vi "Simplex-AO.vi"(3 "Initial Simplex Guess":path=path "C:/Users/Mlodzianoski/Desktop/Microscope 2 Labview Programs/VIs/DM/Mike/FitVal_ZMode_Depth_Corr_April5-2017_Temp.txt", 5 "Current Z":dbl=0.096933, 6 "DM Function":T1=enum."Simplex Correction", 8 "Cycle #":u16, 9 "Step #":u16, 13 "Initial Z":dbl=0.104477, 14 "Use Coverslip Postion":bool=TRUE, 15 "Coverslip Position":dbl=0.103603) -> (19 "Xmin_final":dbl[](array[numeric]))   [LabVIEW 2015]
uses:
  subvis/DM Function_v2.ctl
panel:
  in  "Vertical Coma":bool
  in  "Horizontal Coma":bool
  in  "Vertical Astigmatism":bool
  in  "Oblique Astigmatism":bool
  in  "2nd Spherical Aberration":bool
  in  "1st  Spherical Aberration":bool
  in  "a":dbl=-5e-05 format="%#_13g"
  in  "b":dbl=0.0253 format="%#_13g"
  in  "c":dbl=1.5 format="%#_13g"
  in  "Use Adaptive Astigmatism":bool
  in  "Zernike Modes 3":i32[](array[numeric])
  out "camera sub-readout":u16[][](graph)
  out "current n":i32
  in  "Use Cursor":bool
  in  "boxsize":i32=200
  in  "Use Simplex Results":bool
  in  "Zernike Modes 1":i32[](array[numeric])=[11, 22]
  in  "Zernike Modes 2":i32[](array[numeric])=[5, 6, 7, 8]
  out "Original Simplex Input":dbl[](array[numeric])
  out "Imaging Astigmatism Values":string[](array[string])
  in  "N":i32=40
  out "Tolerance Met":bool
  in  "parray Tolerance\nThreshold":dbl=0.0005
  in  "x input Tolerance\nThreshold":dbl=0.03
  out "xr":dbl[](array[numeric])
  out "parray":dbl[](array[numeric])
  out "Simplex Amplitude":dbl[][](array[numeric])
  in  "indM":i32
  in  "pin":dbl format="%#_13g"
  out "xin":dbl[](array[numeric])
  out "xmax":dbl[](array[numeric])
  out "centroid":dbl[](array[numeric])
  out "xmin":dbl[](array[numeric])
  out "pmax_ind":i32
  out "pmin_ind":i32
  out "psmax":dbl
  out "pmax":dbl
  out "pmin":dbl
  out "pvalr":dbl
  out "camera readout":u16[][](graph)
  # "Adaptive  Astigmatism"
  # "Inputs from \nImaging Program"
  # "Depth Settings"
  # "2nd order polynomial  values from curve fit to data in S. Fig 13"
  # "Aberration Selector"
  # "Column number corresponds to Zernike Mode, value is magnitude of DM."
  # "Current Vertices"
  # "Simplex vertices (updated to show best values)"
  # "Metric pval\ncorresponding \ncurrent set  of \nvertices in \nSimplex \nAmplitude."
  # "Current optimal simplex value"
  # "Final (optimized) simplex values."
  # "Original Simplex Inputs"
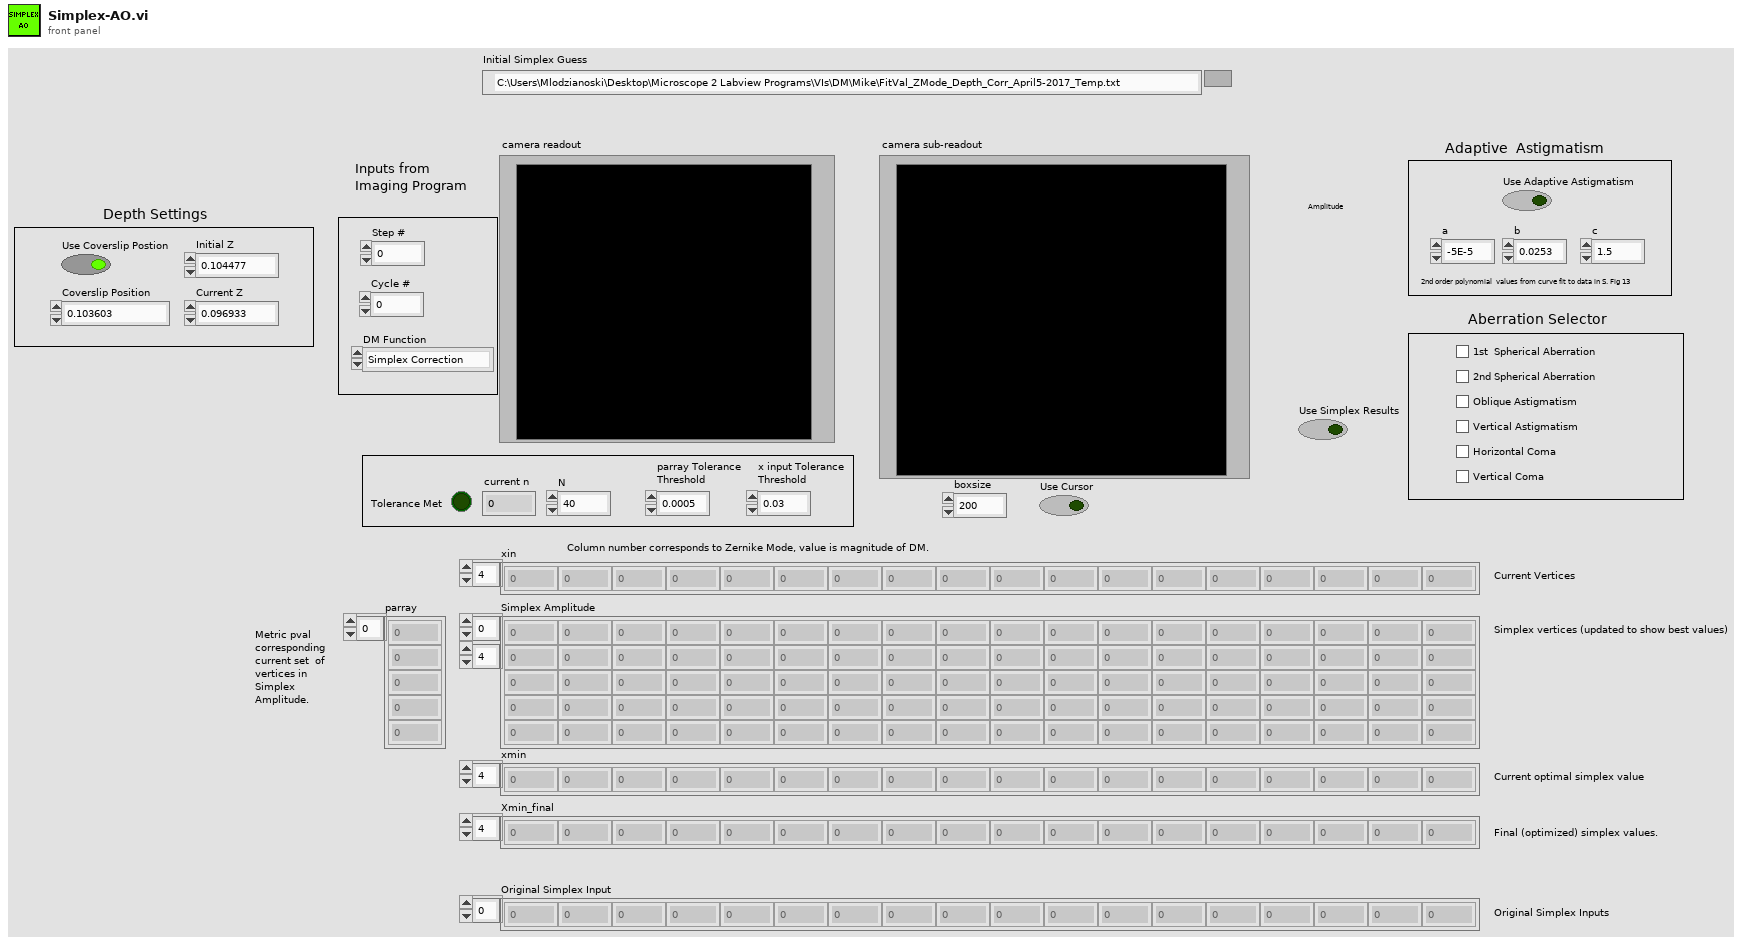
[diagram p1: front panel]
types:
  T1 = typedef "DM Function_v2.ctl" = enum16{"Find Mirror Modes", "Aberration Scan", "Live Aberration Correction", "Idle", "Simplex Correction"}
  T2 = typedef "AbberationControl.ctl" = cluster{"Abberations":dbl[][], "Modes":i32[], "Flat":dbl[], "Abberations ID":string[][]}
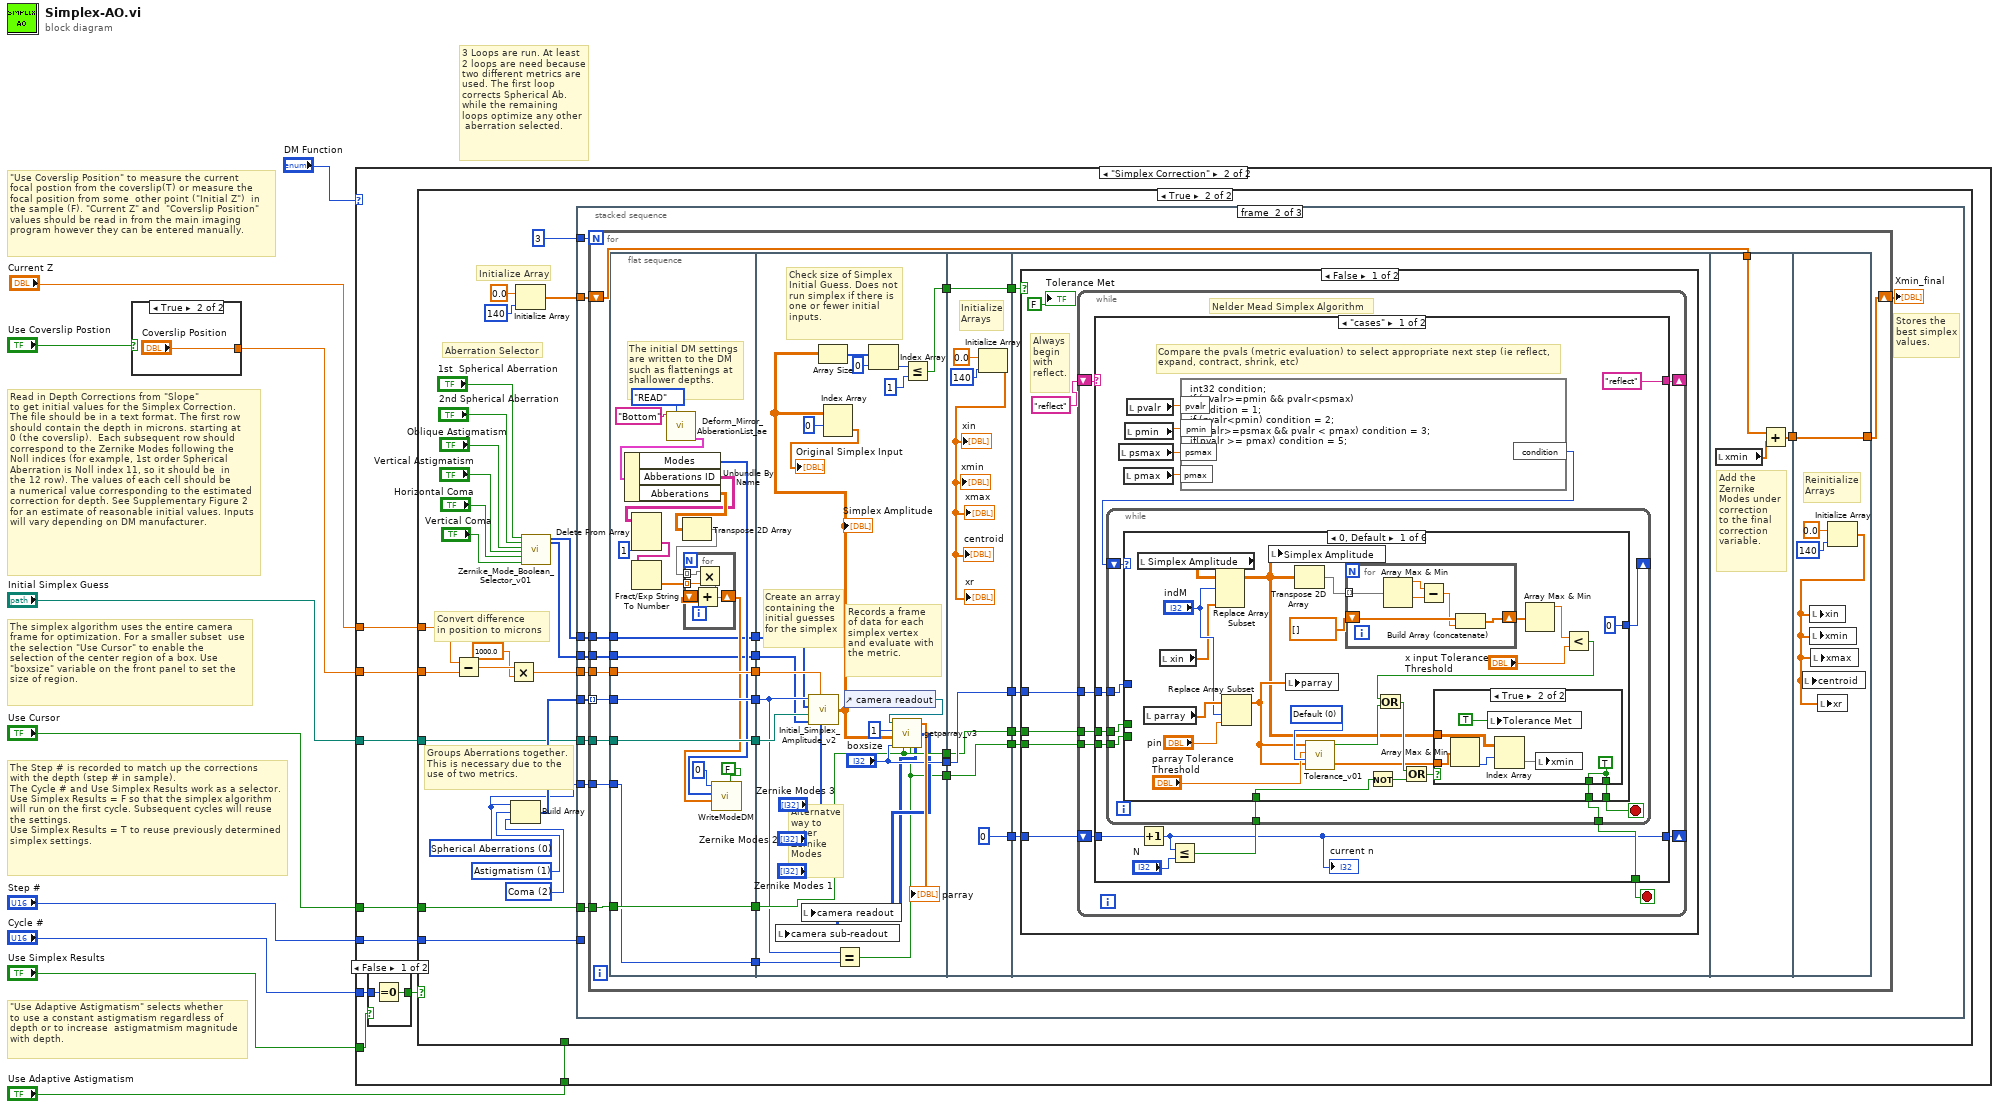
[diagram p0: block diagram]
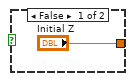
[diagram p2: hidden frame]
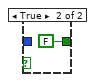
[diagram p4: hidden frame]
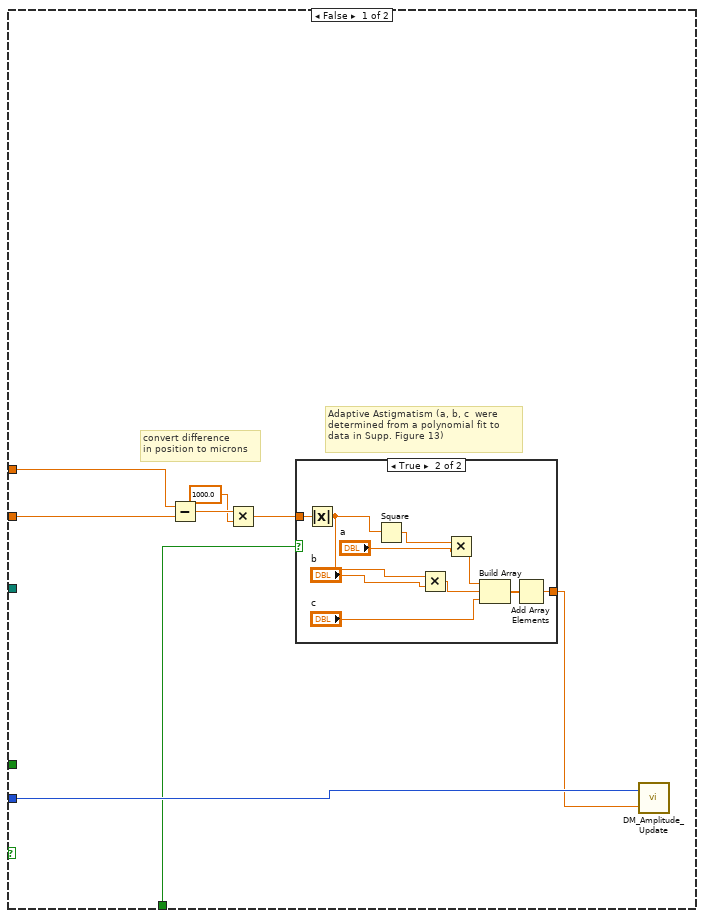
[diagram p5: hidden frame]
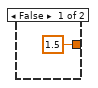
[diagram p6: hidden frame]
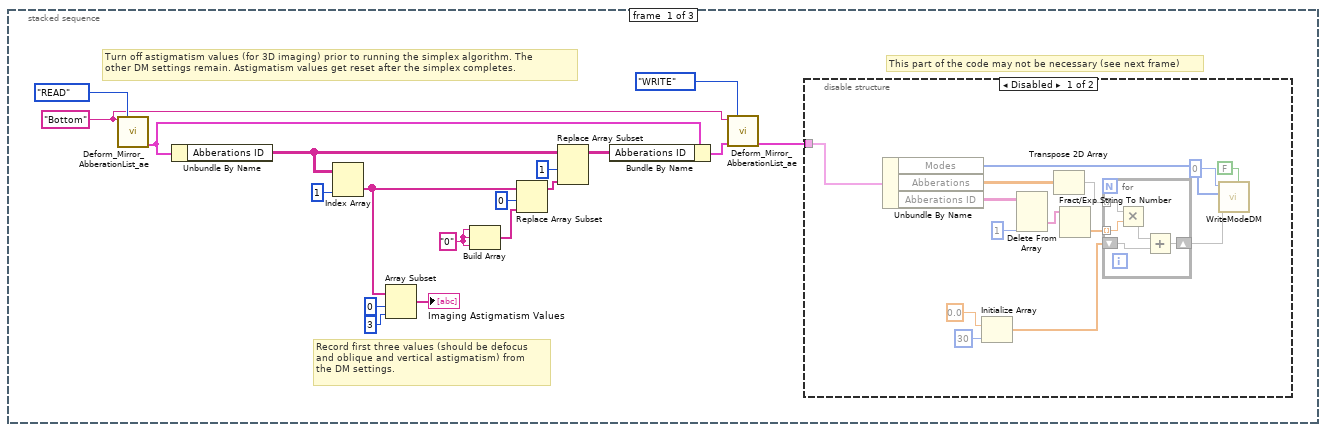
[diagram p7: hidden frame]
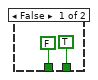
[diagram p9: hidden frame]
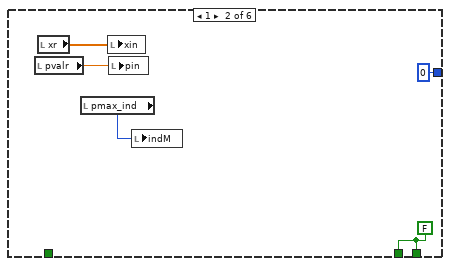
[diagram p10: hidden frame]
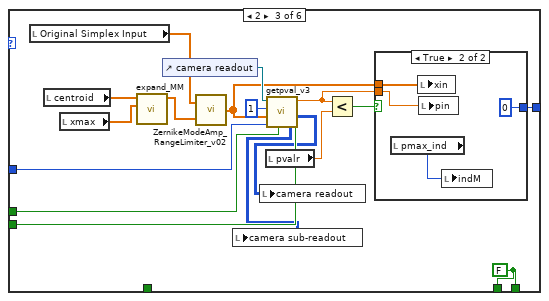
[diagram p11: hidden frame]
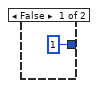
[diagram p12: hidden frame]
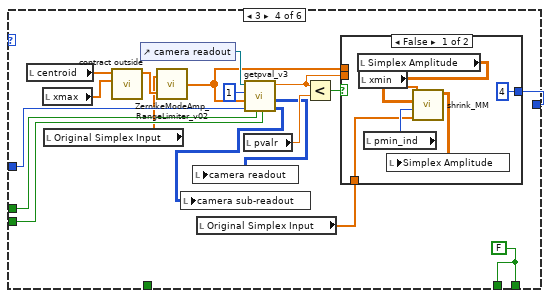
[diagram p13: hidden frame]
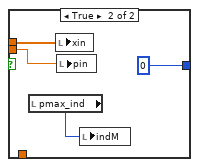
[diagram p14: hidden frame]
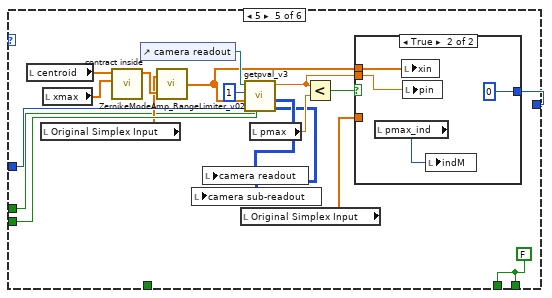
[diagram p15: hidden frame]
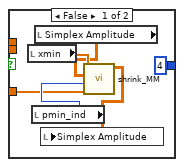
[diagram p16: hidden frame]
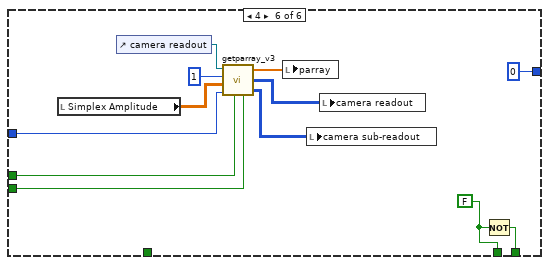
[diagram p17: hidden frame]
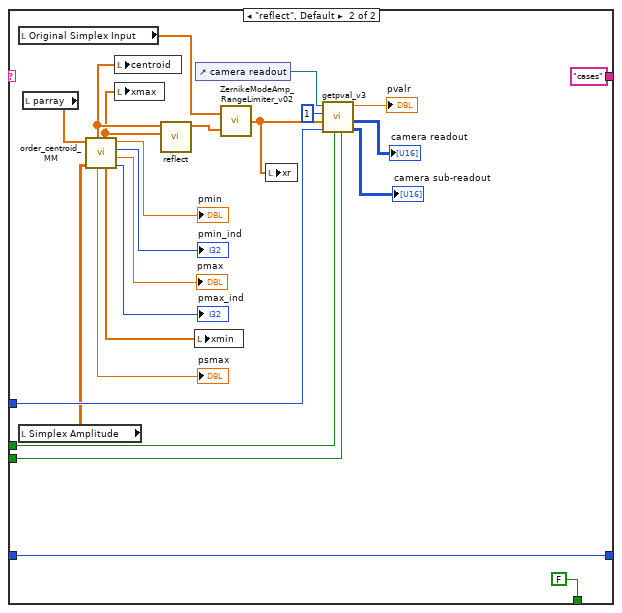
[diagram p18: hidden frame]
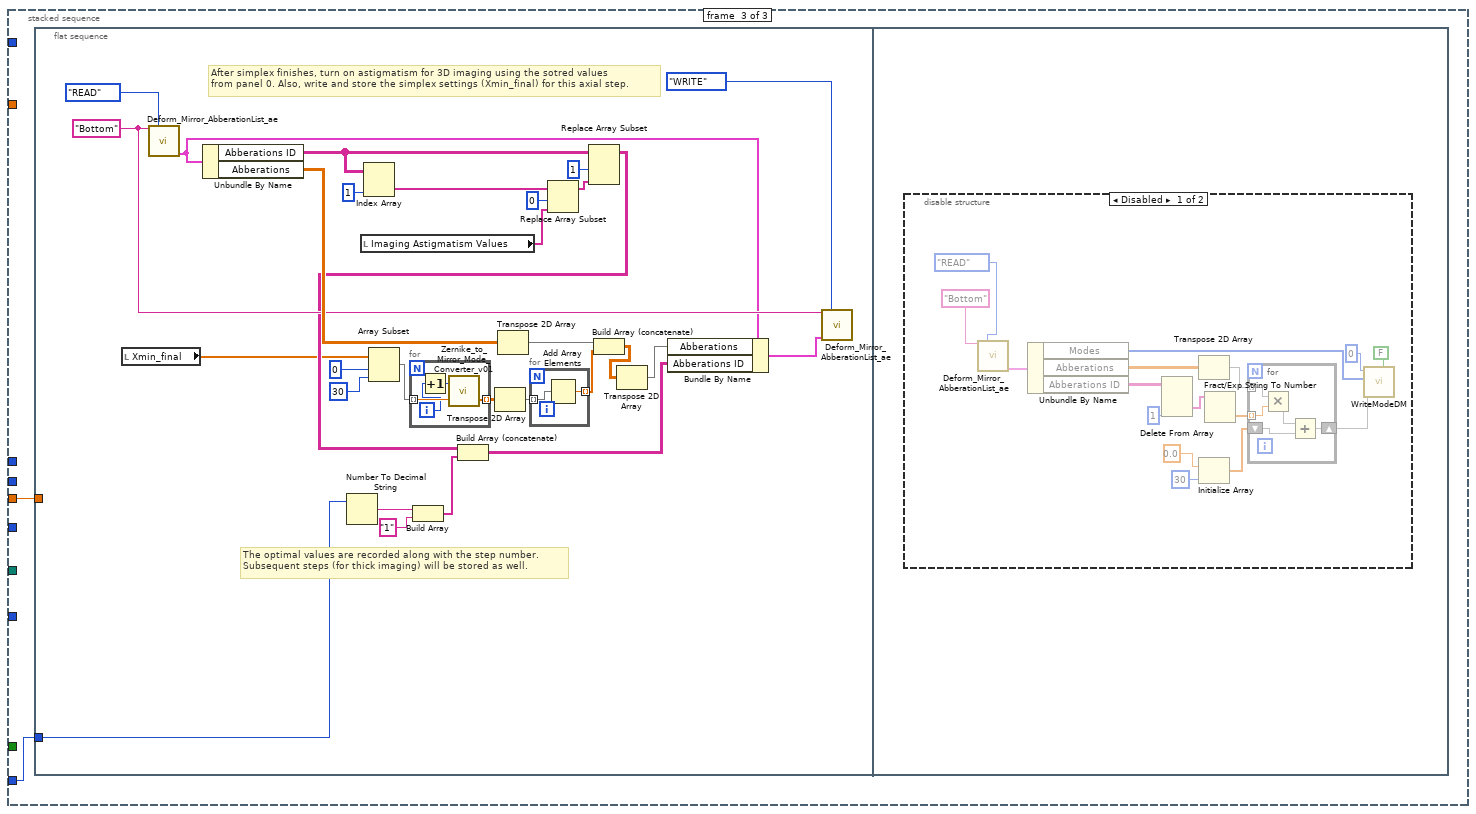
[diagram p20: hidden frame]
diagram:
  # "3 Loops are run. At least\n2 loops are need because\ntwo different metrics are\nused. The first loop \ncorrects Spherical Ab. \nwhile the remaining \nloops optimize any other\n aberration selected."
  # "\"Use Adaptive Astigmatism\" selects whether\nto use a constant astigmatism regardless of \ndepth or to increase  astigmatmism magnitude\nwith depth."
  # "The Step # is recorded to match up the corrections\nwith the depth (step # in sample).\nThe Cycle # and Use Simplex Results work as a selector.\nUse Simplex Results = F so that the simplex algorithm\nwill run on the first cycle. Subsequent cycles will reuse \nthe settings. \nUse Simplex Results = T to reuse previously determined\nsimplex settings."
  # "The simplex algorithm uses the entire camera\nframe for optimization. For a smaller subset  use\nthe selection \"Use Cursor\" to enable the\nselection of the center region of a box. Use\n\"boxsize\" variable on the front panel to set the \nsize of region."
  # "\"Use Coverslip Position\" to measure the current \nfocal postion from the coverslip(T) or measure the\nfocal position from some  other point (\"Initial Z\")  in \nthe sample (F). \"Current Z\" and  \"Coverslip Position\" \nvalues should be read in from the main imaging \nprogram however they can be entered manually."
  # "Read in Depth Corrections from \"Slope\"\nto get initial values for the Simplex Correction.\nThe file should be in a text format. The first row\nshould contain the depth in microns. starting at \n0 (the coverslip).  Each subsequent row should \ncorrespond to the Zernike Modes following the \nNoll indices (for example, 1st order Spherical\nAberration is Noll index 11, so it should be  in \nthe 12 row). The values of each cell should be \na numerical value corresponding to the estimated\ncorrection for depth. See Supplementary Figure 2\nfor an estimate of reasonable initial values. Inputs\nwill vary depending on DM manufacturer."
  n1 = case shown="True" "Use Coverslip Postion" {
    tunnel: ["Initial Z" "Coverslip Position"] -> w10
    frame False {
    }
    frame True {
    }
  }
  n2 = case shown="\"Simplex Correction\"" "DM Function" {
    tunnel: "Current Z" -> [_ w21]
    tunnel: w10 -> [_ w20]
    tunnel: "Initial Simplex Guess" -> [_ w19]
    tunnel: "Step #" -> [_ w18]
    tunnel: "Cycle #" -> [_ w17]
    tunnel: "Use Simplex Results" -> [_ w14]
    tunnel: "Use Cursor" -> [_ w15]
    tunnel: "Use Adaptive Astigmatism" -> [_ w13]
    frame "Idle", Default {
    }
    frame "Simplex Correction" {
      n3 = case shown="False" w14 {
        tunnel: w17 -> [w23 _]
        tunnel: [w22 FALSE] -> w16
        frame False {
          n4 = Equal To 0?(x=w23) -> (x = 0?=w22:bool)
        }
        frame True {
        }
      }
      n5 = case shown="True" w16 {
        tunnel: w21 -> [w28 w65]
        tunnel: w20 -> [w27 w64]
        tunnel: w19 -> [_ w45]
        tunnel: w18 -> [w32 w57]
        tunnel: w15 -> [_ w56]
        tunnel: w13 -> [w26 _]
        frame False {
          # "Adaptive Astigmatism (a, b, c  were\ndetermined from a polynomial fit to \ndata in Supp. Figure 13)"
          # "convert difference \nin position to microns"
          n6 = Subtract(x=w28, y=w27) -> (x-y=w30:dbl)
          n7 = Multiply(x=w30, y=1000.0) -> (x*y=w31:dbl)
          n8 = case shown="True" w26 {
            tunnel: w31 -> [_ w43]
            tunnel: [1.5 ("y") w38] -> w25
            frame False {
            }
            frame True {
              n9 = Absolute Value(x=w43) -> (abs(x)=w41:dbl)
              n10 = Square(x=w41) -> (x^2=w42:dbl)
              n11 = Multiply(x=w41, y="b") -> (x*y=w37:dbl)
              n12 = Multiply(x=w42, y="a") -> (x*y=w40:dbl)
              n13 = Build Array(w40, w37, "c") -> (w39:dbl[])
              n14 = Add Array Elements(numeric array=w39) -> (sum=w38:dbl)
            }
          }
          n15 = call "DM_Amplitude_Update.vi"("Adaptive Astigmatism Value"=w25, "Step #"=w32) -> ()  [unwired: 1 in]
        }
        frame True {
          w54 = u16 2 items=["Spherical Aberrations", "Astigmatism", "Coma"] ("Aberration Correction Choice")
          w55 = u16 1 items=["Spherical Aberrations", "Astigmatism", "Coma"] ("Aberration Correction Choice")
          w44 = u16 0 items=["Spherical Aberrations", "Astigmatism", "Coma"] ("Aberration Correction Choice")
          # "Groups Aberrations together.\nThis is necessary due to the \nuse of two metrics."
          # "Aberration Selector"
          # "Initialize Array"
          # "Convert difference \nin position to microns"
          n16 = Subtract(x=w65, y=w64) -> (x-y=w67:dbl)
          n17 = Multiply(x=w67, y=1000.0) -> (x*y=w63:dbl)
          n18 = Build Array(w44, w55, w54) -> (w61:u16[])
          n19 = Initialize Array(0.0 ("element"), 140 ("dimension size")) -> (w58:dbl[])
          n20 = call "Zernike_Mode_Boolean_Selector_v01.vi"("1st  Spherical Aberration"="1st  Spherical Aberration", "2nd Spherical Aberration"="2nd Spherical Aberration", "Oblique Astigmatism"="Oblique Astigmatism", "Vertical Astigmatism"="Vertical Astigmatism", "Horizontal Coma"="Horizontal Coma", "Vertical Coma"="Vertical Coma") -> ("ZM 1"=w47:i32[], "ZM 2"=w46:i32[])  [unwired: 12 in]
          n21 = stacked-sequence {
            tunnel: w63 -> [_ w114 w401]
            tunnel: w45 -> [_ w113 _]
            tunnel: 3 -> [_ w112 _]
            tunnel: w58 -> [_ w109 _]
            tunnel: w61 -> [_ w111 _]
            tunnel: w57 -> [_ _ w402]
            tunnel: w56 -> [_ w108 _]
            tunnel: w44 -> [_ w107 _]
            tunnel: w47 -> [_ w106 _]
            tunnel: w46 -> [_ w105 _]
            frame #0 {
              w71 = "0"
              w84 = "Bottom" ("Mirror ID")
              # "This part of the code may not be necessary (see next frame)"
              # "Turn off astigmatism values (for 3D imaging) prior to running the simplex algorithm. The \nother DM settings remain. Astigmatism values get reset after the simplex completes."
              # "Record first three values (should be defocus \nand oblique and vertical astigmatism) from \nthe DM settings."
              n22 = call "Deform_Mirror_AbberationList_ae.vi"("Mirror ID"=w84, "Enum"=enum16{"WRITE", "READ"}."READ") -> ("Abberation Cluster Out"=w81:T2)  [unwired: 12 in, 1 out]
              n23 = Unbundle By Name(w81) -> ("Abberations ID"=w75:string[][])
              n24 = Index Array(array=w75, index (col)=1 ("disabled index (col)")) -> (element=w76:string[])  [unwired: 1 in]
              n25 = Array Subset(array=w76, index=0, length=3) -> (→"Imaging Astigmatism Values":string[])
              n26 = Build Array(w71, w71, w71) -> (w70:string[])
              n27 = Replace Array Subset(array=w76, new element=w70, index=0 ("index (row)")) -> (w74:string[])
              n28 = Replace Array Subset(array=w75, new element=w74, index (col)=1 ("disabled index (col)")) -> (w72:string[][])  [unwired: 1 in]
              n29 = Bundle By Name(cluster=w81, "Abberations ID"=w72) -> (w82:T2)
              n30 = call "Deform_Mirror_AbberationList_ae.vi"("Mirror ID"=w84, "Enum"=enum16{"WRITE", "READ"}."WRITE", "Abberation Cluster In"=w82) -> ("Abberation Cluster Out"=w68:T2)  [unwired: 11 in, 1 out]
              n31 = disable-structure shown="Disabled" {
                disable-tunnel: w68 -> [w89 _]
                frame Disabled {
                  n32 = Unbundle By Name(w89) -> ("Modes"=w92:i32[], "Abberations"=w97:dbl[][], "Abberations ID"=w96:string[][])
                  n33 = Initialize Array(0.0 ("element"), 30 ("dimension size")) -> (w86:dbl[])
                  n34 = Delete From Array(array=w96, index (col)=1 ("index")) -> (deleted portion=w94:string[])  [unwired: 2 in, 1 out]
                  n35 = Transpose 2D Array(2D array=w97) -> (transposed array=w98:dbl[][])
                  n36 = Fract/Exp String To Number(string=w94) -> (number=w99:dbl[])  [unwired: 3 in, 1 out]
                  n37 = for {
                    shift-right: [w100] -> w93
                    shift-left: w86 -> [w102]
                    tunnel: w98 -> [w104] mode=indexing
                    tunnel: w99 -> [w103] mode=indexing
                    n38 = Multiply(x=w104, y=w103) -> (x*y=w101:dbl[])
                    n39 = Add(x=w101, y=w102) -> (x+y=w100:dbl[])
                  }
                  n40 = call "WriteModeDM.vi"("ClearV"=FALSE, "Amplitudes"=w93, "Modes"=w92, "Device"=0) -> ()  [unwired: 7 in, 1 out]
                }
                frame Enabled {
                }
              }
            }
            frame #1 {
              # "Stores the\nbest simplex\nvalues."
              n41 = for {
                N: w112 -> [_]
                tunnel: w114 -> [w140]
                tunnel: w113 -> [w139]
                tunnel: w111 -> [w138] mode=indexing
                shift-right: [w137] -> w110
                shift-left: w109 -> [w131]
                tunnel: w108 -> [w126]
                tunnel: w107 -> [w120]
                tunnel: w106 -> [w117]
                tunnel: w105 -> [w115]
                n42 = flat-sequence {
                  tunnel: w138 -> [w158]
                  tunnel: w139 -> [w159]
                  tunnel: w140 -> [w160]
                  tunnel: [w160] -> w130
                  tunnel: [w159] -> w129
                  tunnel: [w158] -> w128
                  tunnel: [w145] -> w127
                  tunnel: w126 -> [w145]
                  tunnel: [w144] -> w121
                  tunnel: w120 -> [w144]
                  tunnel: [w142] -> w118
                  tunnel: w117 -> [w142]
                  tunnel: [w141] -> w116
                  tunnel: w115 -> [w141]
                  tunnel: [w170] -> w135
                  tunnel: ["boxsize"] -> w133
                  tunnel: w130 -> [w185]
                  tunnel: w129 -> [w184]
                  tunnel: w128 -> [w172]
                  tunnel: w127 -> [w180]
                  tunnel: [w180] -> w124
                  tunnel: [w175] -> w122
                  tunnel: w121 -> [w171]
                  tunnel: w118 -> [w168]
                  tunnel: w116 -> [w167]
                  tunnel: w135 -> [w196]
                  tunnel: [w196] -> w134
                  tunnel: w133 -> [w195]
                  tunnel: [w195] -> w132
                  tunnel: [w191] -> w125
                  tunnel: w124 -> [w191]
                  tunnel: [w190] -> w123
                  tunnel: w122 -> [w190]
                  tunnel: [0] -> w119
                  tunnel: w134 -> [w201]
                  tunnel: w132 -> [w200]
                  tunnel: w125 -> [w199]
                  tunnel: w123 -> [w198]
                  tunnel: w119 -> [w197]
                  tunnel: w131 -> [w394]
                  tunnel: [w395] -> w136
                  tunnel: [w400] -> w137
                  tunnel: w136 -> [w400]
                  frame #0 {
                    # "The initial DM settings\nare written to the DM\nsuch as flattenings at \nshallower depths."
                    n43 = call "Deform_Mirror_AbberationList_ae.vi"("Mirror ID"="Bottom", "Enum"=enum16{"WRITE", "READ"}."READ") -> ("Abberation Cluster Out"=w155:T2)  [unwired: 12 in, 1 out]
                    n44 = Unbundle By Name(w155) -> ("Modes"=w146:i32[], "Abberations ID"=w149:string[][], "Abberations"=w150:dbl[][])
                    n45 = Delete From Array(array=w149, index (col)=1 ("index")) -> (deleted portion=w153:string[])  [unwired: 2 in, 1 out]
                    n46 = Fract/Exp String To Number(string=w153) -> (number=w154:dbl[])  [unwired: 3 in, 1 out]
                    n47 = Transpose 2D Array(2D array=w150) -> (transposed array=w151:dbl[][])
                    n48 = for {
                      shift-right: [w163] -> w147
                      shift-left: _ -> [w165]
                      tunnel: w151 -> [w162] mode=indexing
                      tunnel: w154 -> [w161] mode=indexing
                      n49 = Multiply(x=w162, y=w161) -> (x*y=w164:dbl[])
                      n50 = Add(x=w164, y=w165) -> (x+y=w163:dbl[])
                    }
                    n51 = call "WriteModeDM.vi"("ClearV"=FALSE, "Amplitudes"=w147, "Modes"=w146, "Device"=0) -> ()  [unwired: 7 in, 1 out]
                  }
                  frame #1 {
                    # "Alternatve\nway to \nenter \nZernike\nModes"
                    # "Records a frame\nof data for each \nsimplex vertex \nand evaluate with \nthe metric."
                    # "Check size of Simplex \nInitial Guess. Does not\nrun simplex if there is  \none or fewer initial\ninputs."
                    # "Create an array\ncontaining the \ninitial guesses \nfor the simplex"
                    n52 = call "Initial_Simplex_Amplitude_v2.vi"("Zernike Modes 3"="Zernike Modes 3", "Depth (um)"=w185, "Zernike Modes 2"=w167, "Slope"=w184, "Zernike Modes 1"=w168, "Aberration Correction Choice"=w172) -> ("Initial Simplex Amplitude"=w166:dbl[][])
                    "Simplex Amplitude" <- w166
                    n53 = Array Size(array=w166) -> (size(s)=w179:i32[])
                    n54 = Index Array(array=w166, index (row)=0) -> (element=→"Original Simplex Input":dbl[])  [unwired: 1 in]
                    n55 = Equal?(x=w172, y=w171) -> (x = y?=w170:bool)
                    n56 = control-ref of="camera readout"() -> (w186:refnum<vi>)
                    n57 = Index Array(array=w179, index=0) -> (element=w177:i32)
                    n58 = call "getparray_v3.vi"("IntensityGraph in"=w186, "Metric Choice"=w170, "Frames number"=1, "update M"=w166, "Use Cursor"=w180, "boxsize"="boxsize") -> ("Array"=→"parray":dbl[], "subarray"=w174:u16[][], "sub subarray"=w173:u16[][])
                    n59 = local write "camera sub-readout"(w173) -> ()
                    n60 = local write "camera readout"(w174) -> ()
                    n61 = Less Or Equal?(x=w177, y=1) -> (x <= y?=w175:bool)
                  }
                  frame #2 {
                    # "Initialize\nArrays"
                    n62 = Initialize Array(0.0 ("element"), 140 ("dimension size")) -> (→"centroid" →"xmax" →"xmin" →"xr" →"xin":dbl[])
                  }
                  frame #3 {
                    n63 = case shown="False" w198 {
                      tunnel: w201 -> [w206 _]
                      tunnel: w200 -> [w205 _]
                      tunnel: w199 -> [w204 _]
                      tunnel: w197 -> [w203 _]
                      frame False {
                        # "Always\nbegin \nwith\nreflect."
                        n64 = while {
                          shift-right: [w212] -> _
                          shift-left: "reflect" -> [w215]
                          tunnel: w205 -> [w214]
                          tunnel: w206 -> [w213]
                          tunnel: w204 -> [w210]
                          shift-right: [w208] -> _
                          shift-left: w203 -> [w209]
                          stop <- w211 stop-if-true
                          # "Nelder Mead Simplex Algorithm"
                          n65 = case shown="\"cases\"" w215 {
                            tunnel: w214 -> [w223 w390]
                            tunnel: w213 -> [w222 w389]
                            tunnel: ["reflect" "cases"] -> w212
                            tunnel: [w221 FALSE] -> w211
                            tunnel: w210 -> [w220 w372]
                            tunnel: w209 -> [w217 w370]
                            tunnel: [w216 w370] -> w208
                            frame "cases" {
                              # "Compare the pvals (metric evaluation) to select appropriate next step (ie reflect, \nexpand, contract, shrink, etc)"
                              n66 = local read "psmax"() -> (w227:dbl)
                              n67 = local read "pmax"() -> (w226:dbl)
                              n68 = local read "pmin"() -> (w228:dbl)
                              n69 = local read "pvalr"() -> (w229:dbl)
                              n70 = Increment(x=w217) -> (x+1=w216:i32)
                              "current n" <- w216
                              n71 = Less Or Equal?(x=w216, y="N") -> (x <= y?=w218:bool)
                              n72 = formula code="int32 condition;\nif (pvalr>=pmin && pvalr<psmax)\n condition = 1;\nif (pvalr<pmin) condition = 2;\nif(pvalr>=psmax && pvalr < pmax) condition = 3;\nif(pvalr >= pmax) condition = 5;"("pvalr"=w229, "pmin"=w228, "psmax"=w227, "pmax"=w226) -> ("condition"=w225:i32)
                              n73 = while {
                                tunnel: w223 -> [w236]
                                tunnel: w222 -> [w235]
                                shift-right: [w234] -> _
                                shift-left: w225 -> [w237]
                                tunnel: [w231] -> w221
                                tunnel: w218 -> [w232]
                                tunnel: w220 -> [w230]
                                stop <- w233 stop-if-true
                                n74 = case shown="0, Default" w237 {
                                tunnel: w236 -> [_ _ w294 w313 w341 w368]
                                tunnel: w235 -> [_ _ w291 w312 w340 w366]
                                tunnel: [0 0 w288 w308 w336 0] -> w234
                                tunnel: [w247 w275 w285 w307 w335 w363] -> w233
                                tunnel: w232 -> [w246 _ _ _ _ _]
                                tunnel: [w242 w275 w285 w307 w335 w362] -> w231
                                tunnel: w230 -> [_ _ w281 w303 w331 w360]
                                frame 0, Default {
                                w254 = u16 0 items=["Default", "Five Best p-values"] ("Ring")
                                n75 = local read "Simplex Amplitude"() -> (w240:dbl[][])
                                n76 = local read "parray"() -> (w258:dbl[])
                                n77 = local read "xin"() -> (w238:dbl[])
                                n78 = Replace Array Subset(array=w240, new element=w238, index (row)="indM") -> (w239:dbl[][])  [unwired: 1 in]
                                n79 = Replace Array Subset(array=w258, new element="pin", index="indM") -> (w241:dbl[])
                                n80 = local write "Simplex Amplitude"(w239) -> ()
                                n81 = local write "parray"(w241) -> ()
                                n82 = Transpose 2D Array(2D array=w239) -> (transposed array=w259:dbl[][])
                                n83 = call "Tolerance_v01.vi"("Ring"=w254, "Tolerance Threshold"="parray Tolerance\nThreshold", "parray"=w241) -> ("Boolean"=w249:bool)  [unwired: 8 in]
                                n84 = for {
                                tunnel: w259 -> [w274] mode=indexing
                                shift-right: [w271] -> w251
                                shift-left: dbl[] [] -> [w270]
                                n85 = Array Max & Min(array=w274) -> (max value=w273:dbl, min value=w272:dbl)  [unwired: 2 out]
                                n86 = Subtract(x=w273, y=w272) -> (x-y=w269:dbl)
                                n87 = Build Array (concatenate)(w270, w269) -> (w271:dbl[])
                                }
                                n88 = Not(x=w246) -> (.not. x?=w245:bool)
                                n89 = Array Max & Min(array=w251) -> (max value=w252:dbl)  [unwired: 3 out]
                                n90 = Less?(x=w252, y="x input Tolerance\nThreshold") -> (x < y?=w248:bool)
                                n91 = Or(x=w248, y=w249) -> (x .or. y?=w244:bool)
                                n92 = Or(x=w244, y=w245) -> (x .or. y?=w243:bool)
                                n93 = case shown="True" w243 {
                                tunnel: w241 -> [_ w266]
                                tunnel: w239 -> [_ w265]
                                tunnel: [TRUE w263] -> w247
                                tunnel: [FALSE w263] -> w242
                                frame False {
                                }
                                frame True {
                                w263 = TRUE
                                n94 = Array Max & Min(array=w266) -> (min index (indices)=w267:i32)  [unwired: 3 out]
                                n95 = local write "Tolerance Met"(TRUE) -> ()
                                n96 = Index Array(array=w265, index (row)=w267) -> (element=w264:dbl[])  [unwired: 1 in]
                                n97 = local write "xmin"(w264) -> ()
                                }
                                }
                                }
                                frame 1 {
                                w275 = FALSE
                                n98 = local read "pvalr"() -> (w278:dbl)
                                n99 = local read "xr"() -> (w277:dbl[])
                                n100 = local read "pmax_ind"() -> (w279:i32)
                                n101 = local write "xin"(w277) -> ()
                                n102 = local write "pin"(w278) -> ()
                                n103 = local write "indM"(w279) -> ()
                                }
                                frame 2 {
                                w285 = FALSE
                                n104 = local read "Original Simplex Input"() -> (w282:dbl[])
                                n105 = local read "centroid"() -> (w296:dbl[])
                                n106 = local read "xmax"() -> (w295:dbl[])
                                n107 = call "expand_MM.vi"("xmax"=w295, "centroid"=w296) -> ("xe"=w287:dbl[])  [unwired: 9 in]
                                n108 = control-ref of="camera readout"() -> (w293:refnum<vi>)
                                n109 = call "ZernikeModeAmp_RangeLimiter_v02.vi"("x_in"=w287, "Base Values"=w282) -> ("x_out"=w284:dbl[])
                                n110 = local read "pvalr"() -> (w290:dbl)
                                n111 = call "getpval_v3.vi"("Use Cursor"=w281, "Metric Choice"=w291, "boxsize"=w294, "amplitude"=w284, "Frames number"=1, "IntensityGraph in"=w293) -> ("sub-subarray"=w280:u16[][], "subarray"=w283:u16[][], "pval"=w286:dbl)  [unwired: 1 out]
                                n112 = local write "camera sub-readout"(w280) -> ()
                                n113 = local write "camera readout"(w283) -> ()
                                n114 = Less?(x=w286, y=w290) -> (x < y?=w289:bool)
                                n115 = case shown="True" w289 {
                                tunnel: [1 0] -> w288
                                tunnel: w284 -> [_ w300]
                                tunnel: w286 -> [_ w299]
                                frame False {
                                }
                                frame True {
                                n116 = local read "pmax_ind"() -> (w298:i32)
                                n117 = local write "xin"(w300) -> ()
                                n118 = local write "pin"(w299) -> ()
                                n119 = local write "indM"(w298) -> ()
                                }
                                }
                                }
                                frame 3 {
                                w307 = FALSE
                                n120 = local read "centroid"() -> (w318:dbl[])
                                n121 = local read "xmax"() -> (w317:dbl[])
                                n122 = local read "Original Simplex Input"() -> (w305:dbl[])
                                n123 = call "contract outside.vi"("xmax"=w317, "centroid"=w318) -> ("xc"=w319:dbl[])  [unwired: 9 in]
                                n124 = control-ref of="camera readout"() -> (w316:refnum<vi>)
                                n125 = call "ZernikeModeAmp_RangeLimiter_v02.vi"("x_in"=w319, "Base Values"=w305) -> ("x_out"=w309:dbl[])
                                n126 = local read "Original Simplex Input"() -> (w304:dbl[])
                                n127 = local read "pvalr"() -> (w314:dbl)
                                n128 = call "getpval_v3.vi"("Use Cursor"=w303, "Metric Choice"=w312, "boxsize"=w313, "amplitude"=w309, "Frames number"=1, "IntensityGraph in"=w316) -> ("sub-subarray"=w302:u16[][], "subarray"=w306:u16[][], "pval"=w310:dbl)  [unwired: 1 out]
                                n129 = local write "camera sub-readout"(w302) -> ()
                                n130 = local write "camera readout"(w306) -> ()
                                n131 = Less?(x=w310, y=w314) -> (x < y?=w311:bool)
                                n132 = case shown="False" w311 {
                                tunnel: [4 0] -> w308
                                tunnel: w309 -> [_ w328]
                                tunnel: w310 -> [_ w327]
                                tunnel: w304 -> [w320 _]
                                frame False {
                                n133 = local read "Simplex Amplitude"() -> (w321:dbl[][])
                                n134 = local read "xmin"() -> (w324:dbl[])
                                n135 = local read "pmin_ind"() -> (w323:i32)
                                n136 = call "shrink_MM.vi"("Base Values"=w320, "pmin_ind"=w323, "update M"=w321, "x1"=w324) -> ("output M"=w322:dbl[][])  [unwired: 7 in]
                                n137 = local write "Simplex Amplitude"(w322) -> ()
                                }
                                frame True {
                                n138 = local read "pmax_ind"() -> (w326:i32)
                                n139 = local write "xin"(w328) -> ()
                                n140 = local write "pin"(w327) -> ()
                                n141 = local write "indM"(w326) -> ()
                                }
                                }
                                }
                                frame 5 {
                                w335 = FALSE
                                n142 = local read "centroid"() -> (w346:dbl[])
                                n143 = local read "Original Simplex Input"() -> (w333:dbl[])
                                n144 = local read "xmax"() -> (w345:dbl[])
                                n145 = call "contract inside.vi"("xmax"=w345, "centroid"=w346) -> ("xc"=w347:dbl[])  [unwired: 9 in]
                                n146 = control-ref of="camera readout"() -> (w344:refnum<vi>)
                                n147 = call "ZernikeModeAmp_RangeLimiter_v02.vi"("x_in"=w347, "Base Values"=w333) -> ("x_out"=w337:dbl[])
                                n148 = local read "Original Simplex Input"() -> (w332:dbl[])
                                n149 = call "getpval_v3.vi"("Use Cursor"=w331, "Metric Choice"=w340, "boxsize"=w341, "amplitude"=w337, "Frames number"=1, "IntensityGraph in"=w344) -> ("sub-subarray"=w330:u16[][], "subarray"=w334:u16[][], "pval"=w338:dbl)  [unwired: 1 out]
                                n150 = local write "camera sub-readout"(w330) -> ()
                                n151 = local write "camera readout"(w334) -> ()
                                n152 = local read "pmax"() -> (w342:dbl)
                                n153 = Less?(x=w338, y=w342) -> (x < y?=w339:bool)
                                n154 = case shown="True" w339 {
                                tunnel: [4 0] -> w336
                                tunnel: w337 -> [_ w356]
                                tunnel: w338 -> [_ w355]
                                tunnel: w332 -> [w348 _]
                                frame False {
                                n155 = local read "xmin"() -> (w352:dbl[])
                                n156 = local read "pmin_ind"() -> (w351:i32)
                                n157 = local read "Simplex Amplitude"() -> (w349:dbl[][])
                                n158 = call "shrink_MM.vi"("Base Values"=w348, "pmin_ind"=w351, "update M"=w349, "x1"=w352) -> ("output M"=w350:dbl[][])  [unwired: 7 in]
                                n159 = local write "Simplex Amplitude"(w350) -> ()
                                }
                                frame True {
                                n160 = local read "pmax_ind"() -> (w354:i32)
                                n161 = local write "xin"(w356) -> ()
                                n162 = local write "pin"(w355) -> ()
                                n163 = local write "indM"(w354) -> ()
                                }
                                }
                                }
                                frame 4 {
                                w362 = FALSE
                                n164 = local read "Simplex Amplitude"() -> (w361:dbl[][])
                                n165 = control-ref of="camera readout"() -> (w367:refnum<vi>)
                                n166 = call "getparray_v3.vi"("IntensityGraph in"=w367, "Metric Choice"=w366, "Frames number"=1, "update M"=w361, "Use Cursor"=w360, "boxsize"=w368) -> ("Array"=w364:dbl[], "subarray"=w359:u16[][], "sub subarray"=w358:u16[][])
                                n167 = local write "parray"(w364) -> ()
                                n168 = local write "camera sub-readout"(w358) -> ()
                                n169 = local write "camera readout"(w359) -> ()
                                n170 = Not(x=w362) -> (.not. x?=w363:bool)
                                }
                                }
                              }
                            }
                            frame "reflect", Default {
                              n171 = local read "Original Simplex Input"() -> (w373:dbl[])
                              n172 = local read "Simplex Amplitude"() -> (w379:dbl[][])
                              n173 = local read "parray"() -> (w380:dbl[])
                              n174 = call "order_centroid_MM.vi"("update M"=w379, "parray"=w380) -> ("pmax_ind"=→"pmax_ind":i32, "pmax"=→"pmax":dbl, "pmin_ind"=→"pmin_ind":i32, "pmin"=→"pmin":dbl, "xmin"=w376:dbl[], "xmax"=w377:dbl[], "psmax"=→"psmax":dbl, "centroid"=w378:dbl[])  [unwired: 2 in]
                              n175 = local write "centroid"(w378) -> ()
                              n176 = local write "xmax"(w377) -> ()
                              n177 = call "reflect.vi"("xmax"=w377, "centroid"=w378) -> ("xr"=w393:dbl[])  [unwired: 9 in]
                              n178 = local write "xmin"(w376) -> ()
                              n179 = control-ref of="camera readout"() -> (w391:refnum<vi>)
                              n180 = call "ZernikeModeAmp_RangeLimiter_v02.vi"("x_in"=w393, "Base Values"=w373) -> ("x_out"=w375:dbl[])
                              n181 = local write "xr"(w375) -> ()
                              n182 = call "getpval_v3.vi"("Use Cursor"=w372, "Metric Choice"=w389, "boxsize"=w390, "amplitude"=w375, "Frames number"=1, "IntensityGraph in"=w391) -> ("sub-subarray"=→"camera sub-readout":u16[][], "subarray"=→"camera readout":u16[][], "pval"=→"pvalr":dbl)  [unwired: 1 out]
                            }
                          }
                        }
                        "Tolerance Met" <- FALSE ("Tolerance Met")
                      }
                      frame True {
                        # "Skips simplex if there are not enough initial guesses for correction."
                      }
                    }
                  }
                  frame #4 {
                    # "Add the \nZernike \nModes under\ncorrection \nto the final\ncorrection \nvariable."
                    n183 = local read "xmin"() -> (w396:dbl[])
                    n184 = Add(x=w394, y=w396) -> (x+y=w395:dbl[])
                  }
                  frame #5 {
                    # "Reinitialize\nArrays"
                    n185 = Initialize Array(0.0 ("element"), 140 ("dimension size")) -> (w399:dbl[])
                    n186 = local write "centroid"(w399) -> ()
                    n187 = local write "xin"(w399) -> ()
                    n188 = local write "xmin"(w399) -> ()
                    n189 = local write "xmax"(w399) -> ()
                    n190 = local write "xr"(w399) -> ()
                  }
                }
              }
              "Xmin_final" <- w110
            }
            frame #2 {
              n191 = flat-sequence {
                tunnel: w402 -> [w409]
                tunnel: w401 -> [_]
                frame #0 {
                  w410 = "Bottom" ("Mirror ID")
                  # "The optimal values are recorded along with the step number. \nSubsequent steps (for thick imaging) will be stored as well."
                  # "After simplex finishes, turn on astigmatism for 3D imaging using the sotred values \nfrom panel 0. Also, write and store the simplex settings (Xmin_final) for this axial step."
                  n192 = local read "Xmin_final"() -> (w403:dbl[])
                  n193 = call "Deform_Mirror_AbberationList_ae.vi"("Mirror ID"=w410, "Enum"=enum16{"WRITE", "READ"}."READ") -> ("Abberation Cluster Out"=w405:T2)  [unwired: 12 in, 1 out]
                  n194 = Unbundle By Name(w405) -> ("Abberations ID"=w414:string[][], "Abberations"=w415:dbl[][])
                  n195 = Number To Decimal String(number=w409) -> (decimal integer string=w408:string)  [unwired: 1 in]
                  n196 = local read "Imaging Astigmatism Values"() -> (w427:string[])
                  n197 = Index Array(array=w414, index (col)=1 ("disabled index (col)")) -> (element=w425:string[])  [unwired: 1 in]
                  n198 = Array Subset(array=w403, index=0, length=30) -> (w422:dbl[])
                  n199 = for {
                    tunnel: w422 -> [w437] mode=indexing
                    tunnel: [w434] -> w421 mode=indexing
                    i -> [w436]
                    n200 = Increment(x=w436) -> (x+1=w435:i32)
                    n201 = call "Zernike_to_Mirror_Mode_Converter_v01.vi"("Zernike Mode Amplitude"=w437, "Zernike Mode"=w435) -> ("Mirror Mode Amplitude"=w434:dbl[])  [unwired: 1 out]
                  }
                  n202 = Build Array(w408, "1" ("element")) -> (w412:string[])
                  n203 = Transpose 2D Array(2D array=w421) -> (transposed array=w420:dbl[][])
                  n204 = Transpose 2D Array(2D array=w415) -> (transposed array=w418:dbl[][])
                  n205 = for {
                    tunnel: w420 -> [w433] mode=indexing
                    tunnel: [w432] -> w419 mode=indexing
                    n206 = Add Array Elements(numeric array=w433) -> (sum=w432:dbl)
                  }
                  n207 = Replace Array Subset(array=w425, new element=w427, index=0 ("index (row)")) -> (w429:string[])
                  n208 = Replace Array Subset(array=w414, new element=w429, index (col)=1 ("disabled index (col)")) -> (w406:string[][])  [unwired: 1 in]
                  n209 = Build Array (concatenate)(w406, w412) -> (w407:string[][])
                  n210 = Build Array (concatenate)(w418, w419) -> (w417:dbl[][])
                  n211 = Transpose 2D Array(2D array=w417) -> (transposed array=w416:dbl[][])
                  n212 = Bundle By Name(cluster=w405, "Abberations"=w416, "Abberations ID"=w407) -> (w404:T2)
                  n213 = call "Deform_Mirror_AbberationList_ae.vi"("Mirror ID"=w410, "Enum"=enum16{"WRITE", "READ"}."WRITE", "Abberation Cluster In"=w404) -> ()  [unwired: 11 in, 2 out]
                }
                frame #1 {
                  n214 = disable-structure shown="Disabled" {
                    frame Disabled {
                      n215 = call "Deform_Mirror_AbberationList_ae.vi"("Mirror ID"="Bottom", "Enum"=enum16{"WRITE", "READ"}."READ") -> ("Abberation Cluster Out"=w443:T2)  [unwired: 12 in, 1 out]
                      n216 = Unbundle By Name(w443) -> ("Modes"=w446:i32[], "Abberations"=w451:dbl[][], "Abberations ID"=w450:string[][])
                      n217 = Delete From Array(array=w450, index (col)=1 ("index")) -> (deleted portion=w448:string[])  [unwired: 2 in, 1 out]
                      n218 = Transpose 2D Array(2D array=w451) -> (transposed array=w452:dbl[][])
                      n219 = Initialize Array(0.0 ("element"), 30 ("dimension size")) -> (w438:dbl[])
                      n220 = Fract/Exp String To Number(string=w448) -> (number=w453:dbl[])  [unwired: 3 in, 1 out]
                      n221 = for {
                        shift-right: [w454] -> w447
                        shift-left: w438 -> [w456]
                        tunnel: w452 -> [w458] mode=indexing
                        tunnel: w453 -> [w457] mode=indexing
                        n222 = Multiply(x=w458, y=w457) -> (x*y=w455:dbl[])
                        n223 = Add(x=w455, y=w456) -> (x+y=w454:dbl[])
                      }
                      n224 = call "WriteModeDM.vi"("ClearV"=FALSE, "Amplitudes"=w447, "Modes"=w446, "Device"=0) -> ()  [unwired: 7 in, 1 out]
                    }
                    frame Enabled {
                    }
                  }
                }
              }
            }
          }
        }
      }
    }
  }
